vi "test String to Boolean.vi"(11 "Test Case In":refnum<class "test Electronic Datasheet.lvclass">) -> (0 "error out":errorcluster, 3 "Test Case Out":refnum<class "test Electronic Datasheet.lvclass">)   [LabVIEW 2024, in "Test Utilities.lvclass"]
uses:
  Test Utilities.lvclass
  Test Utilities.lvclass/Test Utilities.ctl
  EDS-File-Viewer/Tests/source/test Electronic Datasheet/test Electronic Datasheet.lvclass
  source/CANopen.lvlib
  <vilib>/Astemes/LUnit/Test Case.lvclass
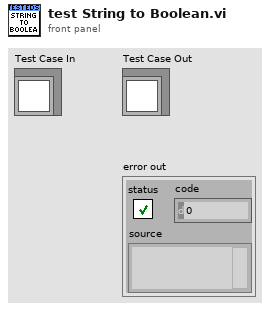
[diagram p1: front panel]
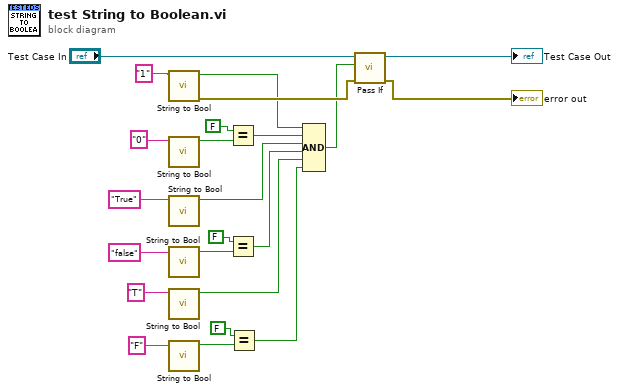
[diagram p0: block diagram]
diagram:
  n1 = call "String to Bool.vi"("Integer String"="1" ("String")) -> ("error out"=w19:errorcluster, "Bool"=w18:bool)  [unwired: 9 in]
  n2 = call "String to Bool.vi"("Integer String"="0" ("String")) -> ("Bool"=w16:bool)  [unwired: 9 in, 1 out]
  n3 = call "String to Bool.vi"("Integer String"="True" ("String")) -> ("Bool"=w4:bool)  [unwired: 9 in, 1 out]
  n4 = call "String to Bool.vi"("Integer String"="false" ("String")) -> ("Bool"=w8:bool)  [unwired: 9 in, 1 out]
  n5 = call "String to Bool.vi"("Integer String"="T") -> ("Bool"=w2:bool)  [unwired: 9 in, 1 out]
  n6 = call "String to Bool.vi"("Integer String"="F") -> ("Bool"=w6:bool)  [unwired: 9 in, 1 out]
  n7 = Equal?(x=FALSE, y=w16) -> (x = y?=w13:bool)
  n8 = Equal?(x=FALSE, y=w8) -> (x = y?=w3:bool)
  n9 = Equal?(x=FALSE, y=w6) -> (x = y?=w1:bool)
  n10 = Compound Arithmetic op=AND(w18, w13, w4, w3, w2, w1) -> (w14:bool)
  n11 = call <vilib>:"Pass If.vi"("error in (no error)"=w19, "Pass?"=w14, "LUnit Test Case In"="Test Case In") -> ("error out"=→"error out":errorcluster, "LUnit Test Case Out"=→"Test Case Out":refnum<class "test Electronic Datasheet.lvclass">)  [unwired: 7 in]
